vi "add_duration.vi"   [LabVIEW 2012]
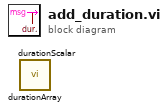
[diagram p0: block diagram]
diagram:
  n1 = call <userlib>:"durationArray.vi"() -> ()  [unwired: 5 in, 1 out]
  n2 = call <userlib>:"durationScalar.vi"() -> ()  [unwired: 5 in, 1 out]
